vi "Swerve Drive Controller.vi"(8 "error in":errorcluster) -> ()   [LabVIEW 2015]
doc: "This VI executes continuously carrying out the current operation and responding to updates or new operations. It will often contain the timing or control code that is difficult to place directly in TeleOp. This VI generally opens all sensors and motors and isolates the rest of the robot code from knowing how the operations are carried out."
uses:
  Swerve Drive Setpoints.ctl
  Swerve Drive Operations.ctl
  <vilib>/Rock Robotics/WPI/CAN/TalonSRX/WPI_CANTalonSRX_APIControlMode.ctl
  <vilib>/Rock Robotics/WPI/CAN/TalonSRX/WPI_CANTalonSRX_APIFeedbackSelect.ctl
  <vilib>/Utility/config.llb/Read Key (Double).vi
  Swerve Drive Published Globals.vi
  <vilib>/Rock Robotics/WPI/MotorControl/WPI_MotorControlOpenCANTalonSRX.vi
  <vilib>/Utility/config.llb/NI_LVConfig.lvlib
panel:
  out "Offsets":dbl[](array[numeric])
  in  "Speed PID":cluster{"P":dbl, "I":dbl, "D":dbl}={"P"=48.0, "I"=0.0, "D"=638.0}
  in  "Ramp Rate":dbl=50.0
  in  "Steering PID":cluster{"P":dbl, "I":dbl, "D":dbl}={"P"=0.0275, "I"=0.000115, "D"=0.682955}
  out "Current\nCmd":string
  # "Tip: It may be helpful to observe inputs and sensor values.\nYou may also want to display tuning or debugging controls."
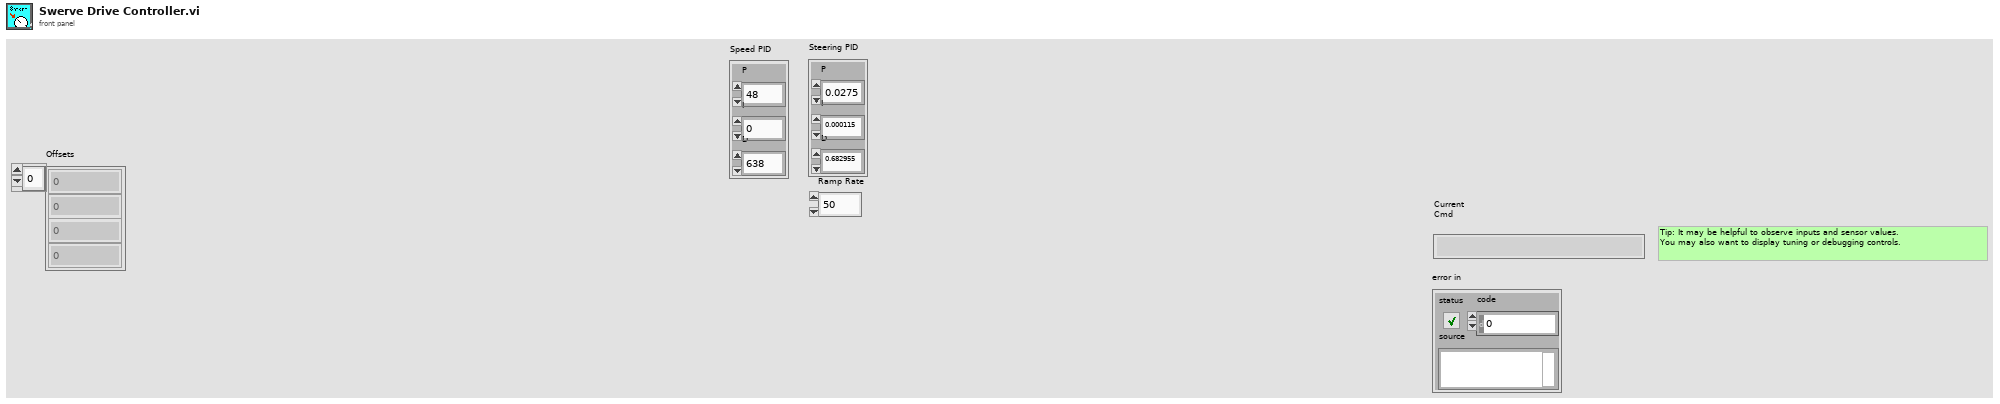
[diagram p1: front panel]
types:
  T1 = typedef "Swerve Drive Setpoints.ctl" = cluster{"Operation":T2, "Duration":dbl, "Joystick":cluster{"Trigger Axes":cluster{"Left":dbl, "Right":dbl}, "Strafe Joystick Axes":cluster{"X":dbl, "Y":dbl}, "Face Joystick Axes":cluster{"X":dbl, "Y":dbl}}, "Position":cluster{"X":dbl, "Y":dbl, "R":dbl}, "Speed Multiplier":dbl}
  T2 = typedef "Swerve Drive Operations.ctl" = enum16{"Reserve", "Read Current", "Immeditate", "Drive", "Go to Coordinates"}
  T3 = typedef "NI_LVConfig.lvlib/Config Data RefNum.ctl" = refnum<k1>
  T4 = typedef "WPI_CANTalonSRX_APIControlMode.ctl" = enum8{"Percent VBus", "Speed", "Position", "Slave", "Unchanged / Invalid", "Voltage Compensation", "Current"}
  T5 = typedef "WPI_CANTalonSRX_APIFeedbackSelect.ctl" = enum16{"Digital Quadrature Encoder", "Analog Potentiometer", "Analog Encoder", "Count on Quad-A (Rising-Edge)", "Count on Quad-A (Falling-Edge)", "CTR Magnetic Enc (Absolute)", "CTR Magnetic Enc (Relative)", "Pulse Width"}
  T6 = typedef "WPI_MotorControlDeviceRef.ctl" = cluster{"DeviceStatus":errorcluster, "Type":T7, "PWM":cluster{"PWM Channel":T8, "DeadBand":T9}, "CAN":cluster{"Device Number":u8, "Control Mode":T10, "Semaphore":T11, "Max Vout":dbl, "TalonSRX Control Mode":T4}, "Invert":bool}
  T7 = typedef "WPI_MotorControlType.ctl" = enum16{"PWM", "CAN", "CANTalonSRX"}
  T8 = typedef "FPGA_DIOPWMChannel.ctl" = enum8{"PWM 0", "PWM 1", "PWM 2", "PWM 3", "PWM 4", "PWM 5", "PWM 6", "PWM 7", "PWM 8", "PWM 9", "PWM MXP 0", "PWM MXP 1", "PWM MXP 2", "PWM MXP 3", "PWM MXP 4", "PWM MXP 5", "PWM MXP 6", "PWM MXP 7", "PWM MXP 8", "PWM MXP 9", "Invalid"}
  T9 = typedef "WPI_PWMDeadband.ctl" = cluster{"Name":string, "maxPositivePwm":i32, "minPositivePwm":i32, "centerPwm":i32, "maxNegativePwm":i32, "minNegativePwm":i32, "angularRange":u16}
  T10 = typedef "WPI_CANJaguar_ControlMode.ctl" = enum8{"Percent VBus", "Current", "Speed", "Position", "Voltage"}
  T11 = typedef "Semaphore RefNum" = refnum<k1>
  T12 = typedef "Command Status Info.ctl" = cluster{"Name":string, "Status":T13, "notifier out":T14}
  T13 = typedef "Completion Status.ctl" = enum16{"Successful", "Aborted", "Incomplete"}
  T14 = typedef "Completion Notifier.ctl" = refnum<notifier>
  T15 = cluster{"Default Command":T1, "Command Timing":cluster{"Start Time (ms)":u32, "Iterations":i32}, "Command Arguments":cluster{"Command Info":T12, "Description":string, "Default Command":T1, "notifier out":refnum<notifier>, "Subsystem Name":string}}
  T16 = cluster{"Trigger Axes":cluster{"Left":dbl, "Right":dbl}, "Strafe Joystick Axes":cluster{"X":dbl, "Y":dbl}, "Face Joystick Axes":cluster{"X":dbl, "Y":dbl}}
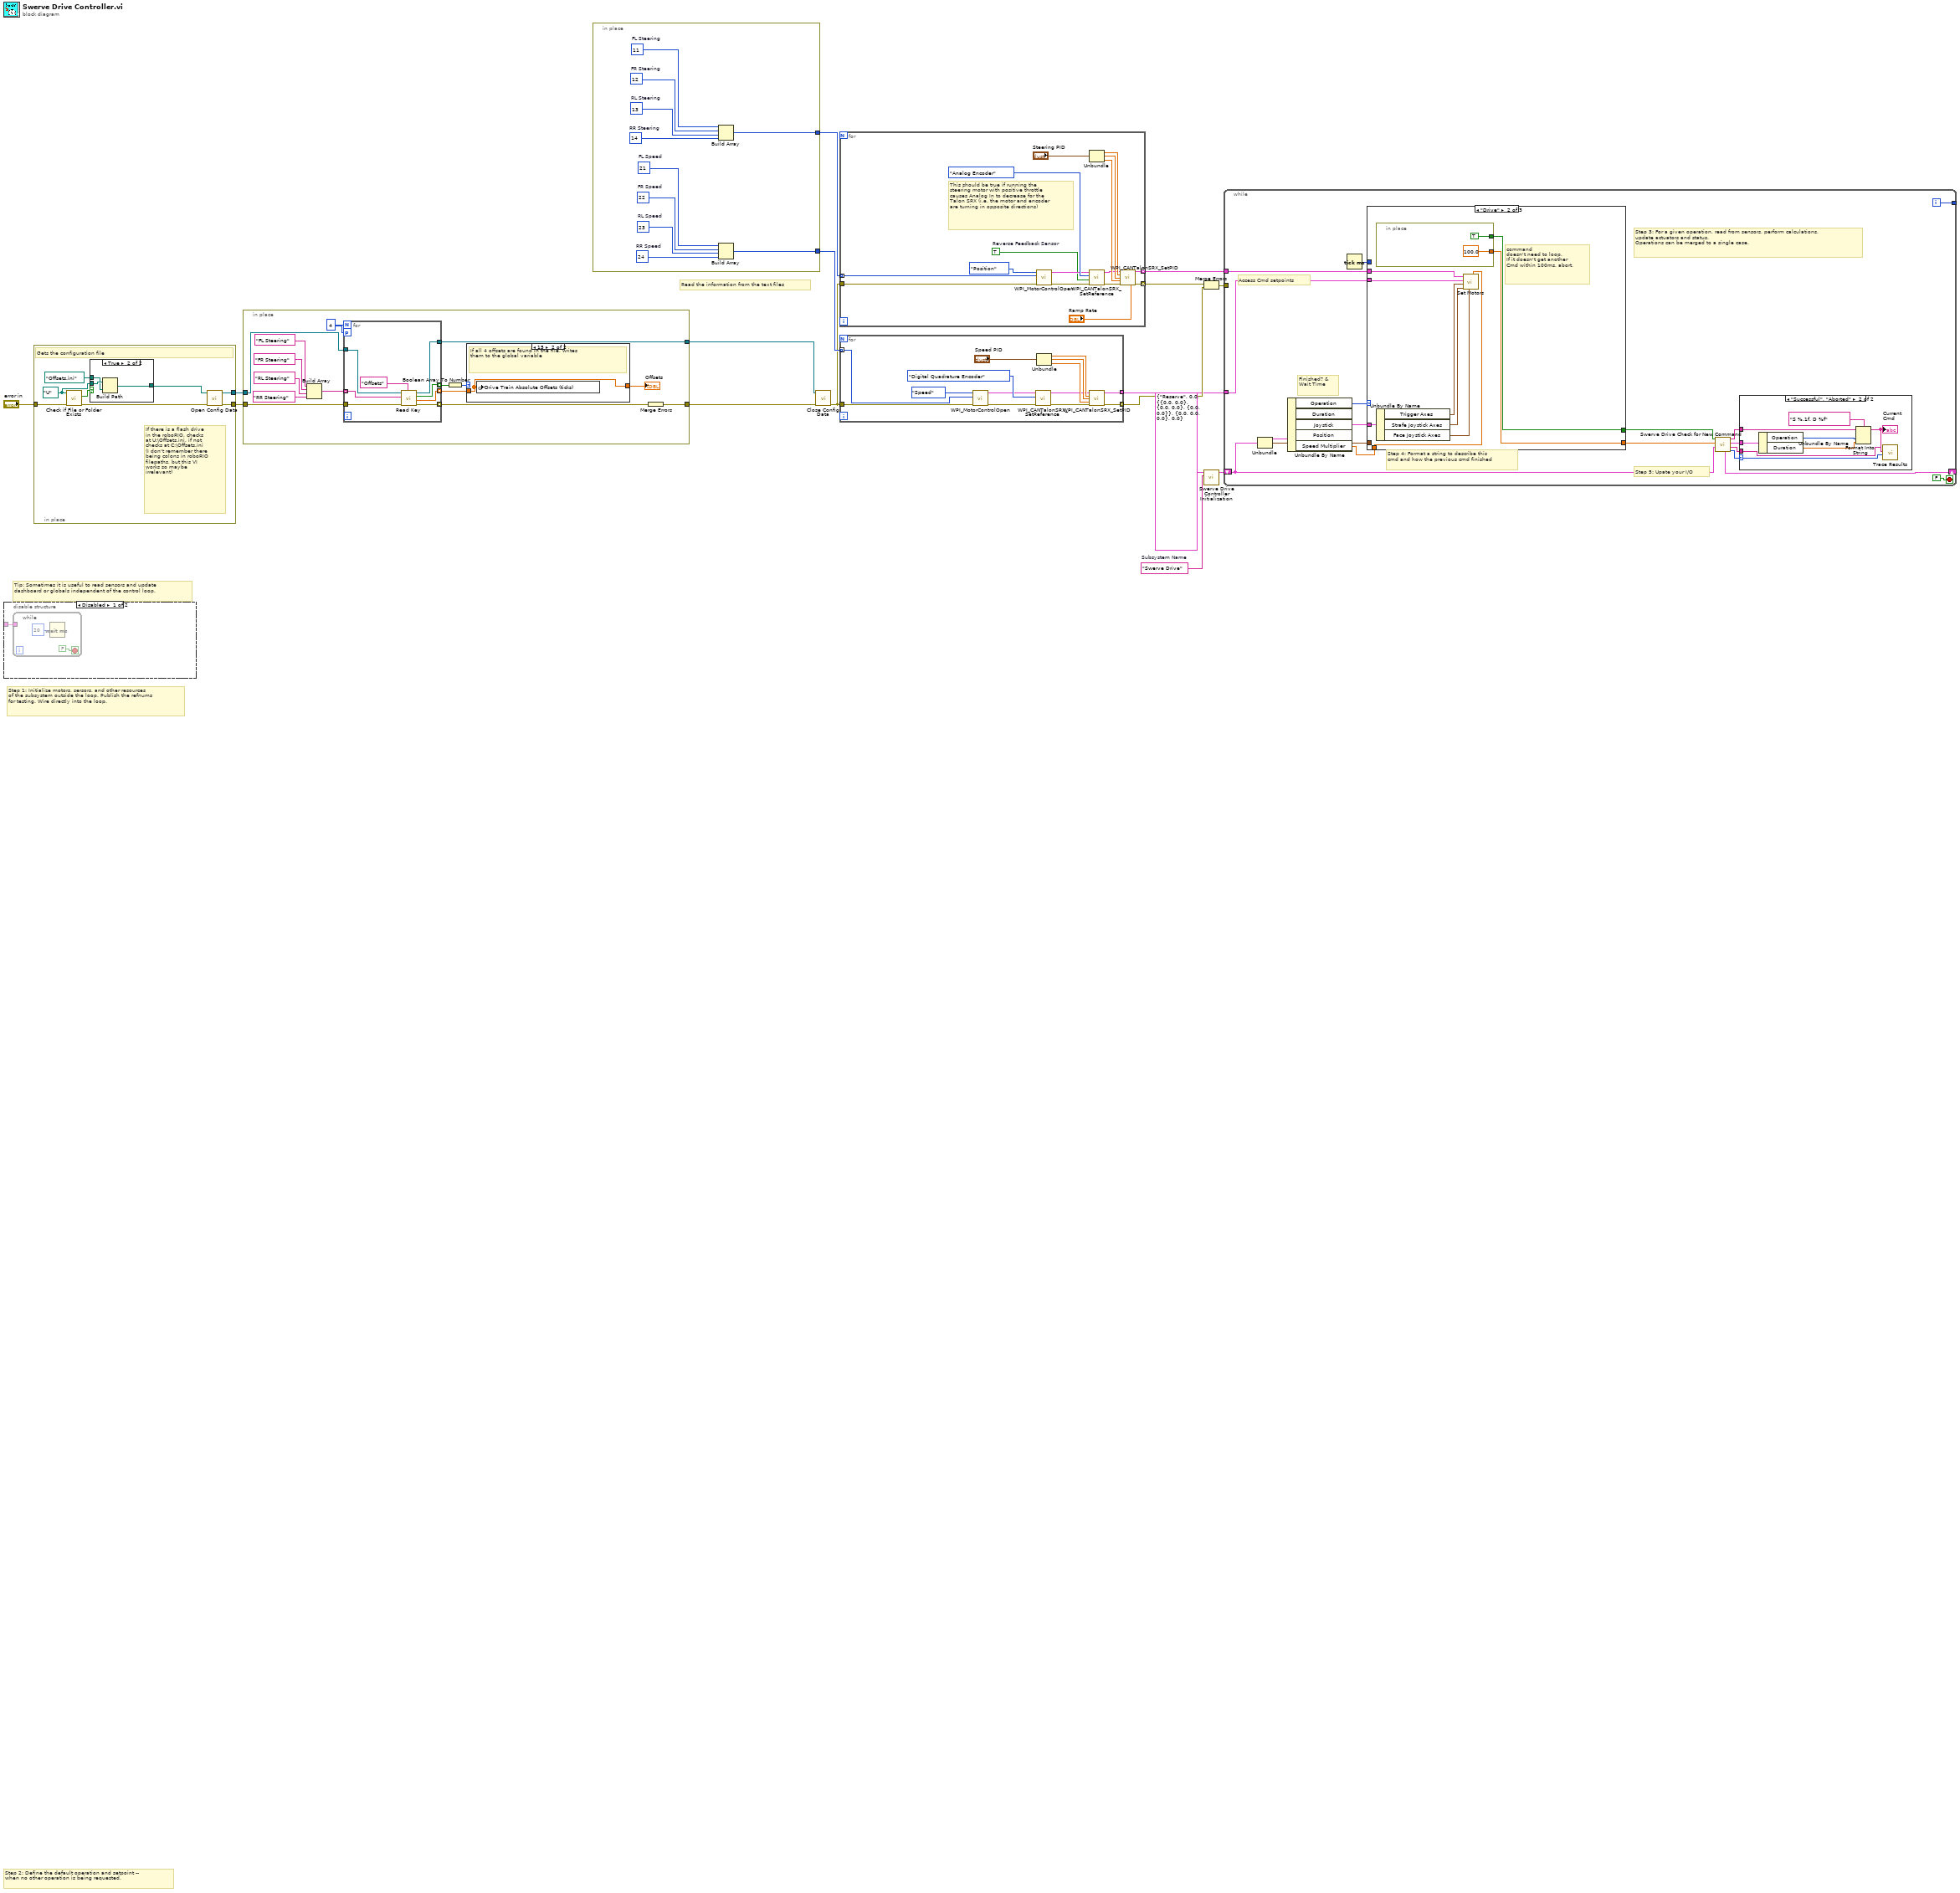
[diagram p0: block diagram]
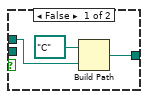
[diagram p2: hidden frame]
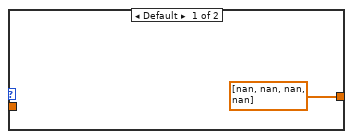
[diagram p3: hidden frame]
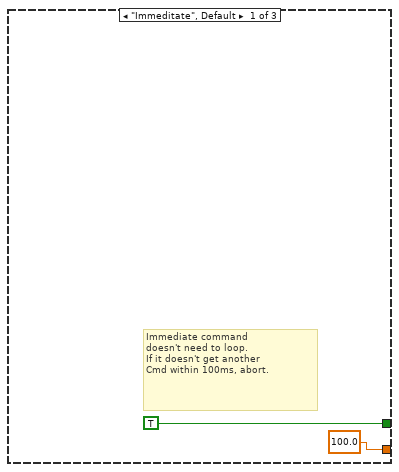
[diagram p6: hidden frame]
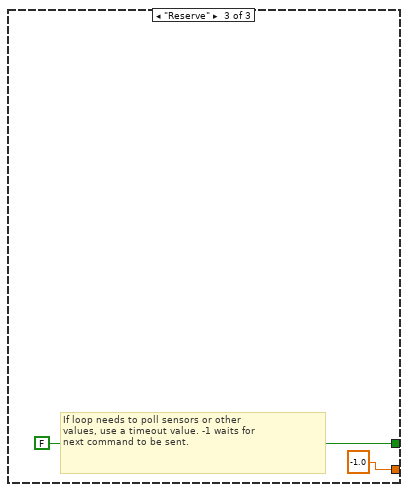
[diagram p7: hidden frame]
diagram:
  w15 = "Swerve Drive"  # Subsystem Name
  # "Read the information from the text files"
  # "Tip: Sometimes it is useful to read sensors and update\ndashboard or globals independent of the control loop."
  # "Step 2: Define the default operation and setpoint --\nwhen no other operation is being requested."
  # "Step 1: Initialize motors, sersors, and other resources\nof the subsystem outside the loop. Publish the refnums\nfor testing. Wire directly into the loop."
  n1 = disable-structure shown="Disabled" {
    disable-tunnel: _ -> [w17 _]
    frame Disabled {
      n2 = while {
        tunnel: w17 -> [_]
        stop <- FALSE stop-if-true
        n3 = Wait (ms)(milliseconds to wait=u32 20) -> ()  [unwired: 1 out]
      }
    }
    frame Enabled {
    }
  }
  n4 = in-place {
    in-place-border: "error in" -> [w27]
    in-place-border: [w25] -> w9
    in-place-border: [w24] -> w8
    w20 = path "U:/" ("base path")
    # "If there is a flash drive\nin the roboRIO, checks\nat U:\\Offsets.ini, if not \nchecks at C:\\Offsets.ini\n(I don't remember there\nbeing colons in roboRIO\nfilepaths, but this VI\nworks so maybe \nirrelevant)"
    # "Gets the configuration file"
    n5 = call <vilib>:"Check if File or Folder Exists.vi"("error in (no error)"=w27, "path"=w20) -> ("error out"=w26:errorcluster, "file or folder exists?"=w21:bool)  [unwired: 7 in, 1 out]
    n6 = case shown="True" w21 {
      tunnel: path "Offsets.ini" ("default name") -> [w30 w31]
      tunnel: [w29 w32] -> w23
      tunnel: w20 -> [_ w33]
      frame False {
        n7 = Build Path(base path=path "C:/", name or relative path=w30) -> (appended path=w29:path)
      }
      frame True {
        n8 = Build Path(base path=w33, name or relative path=w31) -> (appended path=w32:path)
      }
    }
    n9 = call <vilib>:"Open Config Data.vi"("error in (no error)"=w26, "configuration file path"=w23) -> ("error out"=w25:errorcluster, "refnum"=w24:T3)  [unwired: 1 in, 7 out]
  }
  n10 = in-place {
    in-place-border: w9 -> [w38]
    in-place-border: [w36] -> w5
    in-place-border: w8 -> [w37]
    in-place-border: [w34] -> w6
    w48 = 4
    n11 = Build Array("FL Steering", "FR Steering" ("element"), "RL Steering" ("element"), "RR Steering" ("element")) -> (w43:string[])
    n12 = for {
      N: w48 -> [_]
      workers-P: w48 -> [_]
      tunnel: w43 -> [w58] mode=indexing
      tunnel: w37 -> [w57]
      tunnel: [w56] -> w41 mode=indexing
      tunnel: w38 -> [w55]
      tunnel: [w54] -> w42 mode=indexing
      tunnel: [w53] -> w40 mode=indexing
      tunnel: [w52] -> w34
      n13 = call-poly <vilib>:"Read Key.vi"("section"="Offsets", "error in (no error)"=w55, "key"=w58, "refnum"=w57) -> ("error out"=w54:errorcluster, "value"=w56:dbl, "found?"=w53:bool, "refnum out"=w52:T3)  [unwired: 4 in]
    }
    n14 = Boolean Array To Number(Boolean array=w40) -> (number=w39:u32)
    n15 = case shown="15" w39 {
      tunnel: w41 -> [_ w50]
      tunnel: [dbl[] [nan, nan, nan, nan] w50] -> w35
      frame Default {
      }
      frame 15 {
        # "If all 4 offsets are found in the file, writes\nthem to the global variable"
        n16 = global write "Swerve Drive Published Globals.vi" "Drive Train Absolute Offsets (ticks)"(w50) -> ()
      }
    }
    "Offsets" <- w35
    n17 = Merge Errors(w42) -> (w36:errorcluster)
  }
  n18 = in-place {
    in-place-border: [w64] -> w13
    in-place-border: [w59] -> w11
    w68 = u8 11  # FL Steering
    w60 = u8 24  # RR Speed
    w61 = u8 23  # RL Speed
    w62 = u8 22  # FR Speed
    w63 = u8 21  # FL Speed
    w65 = u8 14  # RR Steering
    w66 = u8 13  # RL Steering
    w67 = u8 12  # FR Steering
    n19 = Build Array(w68, w67, w66, w65) -> (w64:u8[])
    n20 = Build Array(w63, w62, w61, w60) -> (w59:u8[])
  }
  n21 = call <vilib>:"Close Config Data.vi"("error in (no error)"=w5, "refnum"=w6) -> ("error out"=w4:errorcluster)  [unwired: 8 in, 1 out]
  n22 = for {
    tunnel: w4 -> [w81]
    tunnel: [w70] -> w12 mode=indexing
    tunnel: w13 -> [w76] mode=indexing
    tunnel: [w69] -> w3 mode=indexing
    w71 = TRUE  # Reverse Feedback Sensor
    # "This should be true if running the\nsteering motor with positive throttle\ncauses Analog In to decrease for the\nTalon SRX (i.e. the motor and encoder\nare turning in opposite directions)"
    n23 = call-poly <vilib>:"WPI_MotorControlOpen.vi"("error in (no error)"=w81, "Device Number"=w76, "Control Mode"=WPI_CANTalonSRX_APIControlMode."Position") -> ("error out"=w77:errorcluster, "MotorControlDeviceRef"=w73:T6)  [unwired: 7 in]
    n24 = Unbundle("Steering PID") -> ("P"=w84:dbl, "I"=w83:dbl, "D"=w82:dbl)
    n25 = call <vilib>:"WPI_CANTalonSRX_SetReference.vi"("error in (no error)"=w77, "Reverse Feedback Sensor"=w71, "Feedback Reference"=WPI_CANTalonSRX_APIFeedbackSelect."Analog Encoder", "CAN Talon SRX Ref"=w73) -> ("error out"=w80:errorcluster, "CAN Talon SRX Ref Out"=w79:T6)  [unwired: 6 in]
    n26 = call <vilib>:"WPI_CANTalonSRX_SetPID.vi"("CAN Talon SRX Ref"=w79, "P"=w84, "I"=w83, "D"=w82, "error in (no error)"=w80, "Ramp Rate"="Ramp Rate") -> ("CAN Talon SRX Ref Out"=w69:T6, "error out"=w70:errorcluster)  [unwired: 8 in]
  }
  n27 = for {
    tunnel: w4 -> [w95]
    tunnel: [w87] -> w14 mode=indexing
    tunnel: w11 -> [w90] mode=indexing
    tunnel: [w86] -> w2 mode=indexing
    n28 = call-poly <vilib>:"WPI_MotorControlOpen.vi"("error in (no error)"=w95, "Device Number"=w90, "Control Mode"=WPI_CANTalonSRX_APIControlMode."Speed") -> ("error out"=w89:errorcluster, "MotorControlDeviceRef"=w88:T6)  [unwired: 7 in]
    n29 = call <vilib>:"WPI_CANTalonSRX_SetReference.vi"("error in (no error)"=w89, "Feedback Reference"=WPI_CANTalonSRX_APIFeedbackSelect."Digital Quadrature Encoder", "CAN Talon SRX Ref"=w88) -> ("error out"=w93:errorcluster, "CAN Talon SRX Ref Out"=w94:T6)  [unwired: 7 in]
    n30 = Unbundle("Speed PID") -> ("P"=w98:dbl, "I"=w97:dbl, "D"=w96:dbl)
    n31 = call <vilib>:"WPI_CANTalonSRX_SetPID.vi"("CAN Talon SRX Ref"=w94, "P"=w98, "I"=w97, "D"=w96, "error in (no error)"=w93) -> ("CAN Talon SRX Ref Out"=w86:T6, "error out"=w87:errorcluster)  [unwired: 9 in]
  }
  n32 = Merge Errors(w12, w14) -> (w10:errorcluster)
  n33 = call "Swerve Drive Controller Initialization.vi"("Subsystem Name"=w15, "Default Command"=T1 {"Operation"=enum."Reserve", "Duration"=0.0, "Joystick"={"Trigger Axes"={"Left"=0.0, "Right"=0.0}, "Strafe Joystick Axes"={"X"=0.0, "Y"=0.0}, "Face Joystick Axes"={"X"=0.0, "Y"=0.0}}, "Position"={"X"=0.0, "Y"=0.0, "R"=0.0}, "Speed Multiplier"=0.0}) -> ("Command Info"=w16:T15)  [unwired: 9 in]
  n34 = while {
    shift-right: [w112] -> _
    shift-left: w16 -> [w103]
    tunnel: [w115] -> _
    tunnel: w10 -> [_]
    tunnel: w3 -> [w105]
    tunnel: w2 -> [w106]
    i -> [w115]
    stop <- FALSE stop-if-true
    # "Step 5: Upate your I/O"
    # "Step 4: Format a string to describe this\ncmd and how the previous cmd finished"
    # "Access Cmd setpoints"
    # "Finished? &\nWait Time"
    # "Step 3: For a given operation, read from sensors, perform calculations,\nupdate actuators and status.\nOperations can be merged to a single case."
    n35 = Unbundle "Unbundle"(w103) -> ("Default Command"=w104:T1, "Command Timing"=w113:cluster{"Start Time (ms)":u32, "Iterations":i32})  [unwired: 1 out]
    n36 = Unbundle By Name(w104) -> ("Operation"=w101:T2, "Joystick"=w100:T16, "Speed Multiplier"=w99:dbl)  [unwired: 2 out]
    n37 = Tick Count (ms)() -> (millisecond timer value=w114:u32)
    n38 = case shown="\"Drive\"" w101 {
      tunnel: [100.0 w134 -1.0] -> w110
      tunnel: [TRUE ("ignore previous (F)") w135 FALSE ("ignore previous (F)")] -> w111
      tunnel: w113 -> [_ _ _]
      tunnel: w114 -> [_ _ _]
      tunnel: w106 -> [_ w130 _]
      tunnel: w105 -> [_ w131 _]
      tunnel: w100 -> [_ w133 _]
      tunnel: w99 -> [_ w127 _]
      frame "Immeditate", Default {
        # "Immediate command\ndoesn't need to loop.\nIf it doesn't get another\nCmd within 100ms, abort."
      }
      frame "Drive" {
        # "command\ndoesn't need to loop.\nIf it doesn't get another\nCmd within 100ms, abort."
        n39 = in-place {
          in-place-border: [TRUE ("ignore previous (F)")] -> w135
          in-place-border: [100.0] -> w134
        }
        n40 = Unbundle By Name(w133) -> ("Trigger Axes"=w132:cluster{"Left":dbl, "Right":dbl}, "Strafe Joystick Axes"=w129:cluster{"X":dbl, "Y":dbl}, "Face Joystick Axes"=w128:cluster{"X":dbl, "Y":dbl})
        n41 = call "Set Motors.vi"("Speed Multipliers"=w127, "Face Joystick Axes"=w128, "Strafe Joystick Axes"=w129, "Trigger Axes"=w132, "Speed Motors"=w130, "Position Motors"=w131) -> ()  [unwired: 5 in, 1 out]
      }
      frame "Reserve" {
        # "If loop needs to poll sensors or other\nvalues, use a timeout value. -1 waits for\nnext command to be sent."
      }
    }
    n42 = call "Swerve Drive Check for New Command.vi"("Current Command"=w103, "Wait time (ms)"=w110, "Finished?"=w111) -> ("Completion"=w107:T13, "Subsystem Name"=w108:string, "Current Command"=w109:T1, "Initial Trace String"=w102:string, "NextCommand"=w112:T15)  [unwired: 4 in]
    n43 = case shown="\"Successful\", \"Aborted\"" w107 {
      selector: w107 -> [_ w124]
      tunnel: w102 -> [_ w120]
      tunnel: w109 -> [_ w121]
      tunnel: w108 -> [_ w117]
      frame "Incomplete", Default {
        # "Continuing current command"
      }
      frame "Successful", "Aborted" {
        # "Report and setup for next command"
        n44 = Unbundle By Name(w121) -> ("Operation"=w123:T2, "Duration"=w118:dbl)
        n45 = Format Into String(format string="S %.1f, D %f", initial string=w120, w123, w118) -> (resulting string=w119:string)  [unwired: 1 in, 1 out]
        "Current\nCmd" <- w119
        n46 = call "Trace Results.vi"("Status of previous command"=w124, "Description"=w119, "Subsystem"=w117) -> ()  [unwired: 9 in]
      }
    }
  }
